vi "TEMPP.vi"() -> ()   [LabVIEW 2017]
panel:
  out "SMOKE ALARM":bool=TRUE
  out "GENERAL ALARM":bool=TRUE
  in  "Smoke Level Set Point":dbl(slide) scale=0.0..100.0
  in  "Smoke Level Detector":dbl(slide) scale=0.0..100.0
  in  "Temp Set Point":dbl(slide) scale=0.0..100.0
  in  "Thermometer":dbl(slide) scale=0.0..100.0
  out "TEMPERATURE ALARM":bool=TRUE
  in  "ON/OFF":bool=TRUE
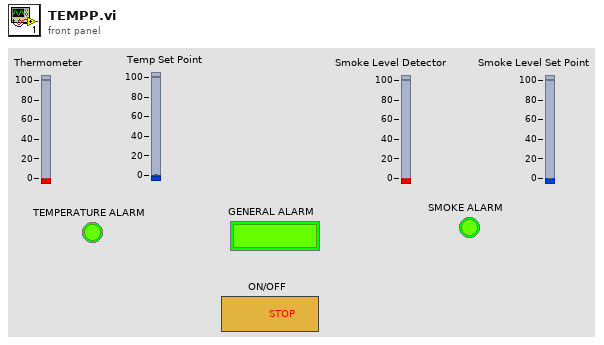
[diagram p1: front panel]
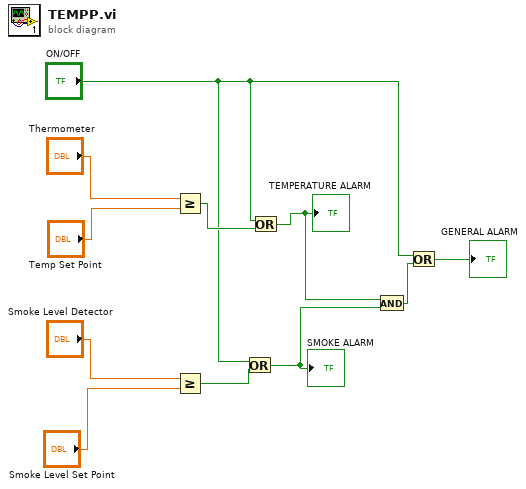
[diagram p0: block diagram]
diagram:
  n1 = Greater Or Equal?(x="Thermometer", y="Temp Set Point") -> (x >= y?=w7:bool)
  n2 = Greater Or Equal?(x="Smoke Level Detector", y="Smoke Level Set Point") -> (x >= y?=w6:bool)
  n3 = Or(x="ON/OFF", y=w6) -> (x .or. y?=w2:bool)
  "SMOKE ALARM" <- w2
  n4 = Or(x="ON/OFF", y=w7) -> (x .or. y?=w3:bool)
  "TEMPERATURE ALARM" <- w3
  n5 = And(x=w3, y=w2) -> (x .and. y?=w5:bool)
  n6 = Or(x="ON/OFF", y=w5) -> (x .or. y?=→"GENERAL ALARM":bool)
